vi "Check Client Computer Namevi.vi"(10 "Computer DNS Name":string, 11 "Name":string) -> ()   [LabVIEW 2025]
uses:
  <vilib>/Rock Robotics/Network Tables/NT Read String.vi
  <vilib>/Rock Robotics/Network Tables/NT Write String.vi
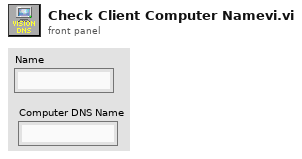
[diagram p1: front panel]
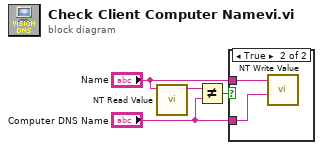
[diagram p0: block diagram]
diagram:
  n1 = call-poly <vilib>:"NT Read Value.vi"("name"="Name") -> ("value"=w2:string)  [unwired: 8 in, 2 out]
  n2 = Not Equal?(x=w2, y="Computer DNS Name") -> (x != y?=w1:bool)
  n3 = case shown="True" w1 {
    tunnel: "Name" -> [_ w6]
    tunnel: "Computer DNS Name" -> [_ w5]
    frame False {
    }
    frame True {
      n4 = call-poly <vilib>:"NT Write Value.vi"("value"=w5, "name"=w6) -> ()  [unwired: 9 in, 1 out]
    }
  }
